vi "ArrDevMeasAction.vi"(6 "Scan":bool, 7 "DevId":i32, 8 "error in (no error)":errorcluster caption="entrée d'erreur (pas d'erreur)", 9 "CurvePointIndex":i32, 10 "AllPointIndex":i32, 11 "Device In":refnum<class "BaseDevice.lvclass"> caption="DNL_LabVIEW Object in") -> (0 "error out":errorcluster caption="sortie d'erreur", 1 "ArrDevDat":T1[](array[typedef]), 2 "ArrDevDatOut":dbl[][](array[numeric]), 3 "Device Out":refnum<class "BaseDevice.lvclass"> caption="DNL_LabVIEW Object out", 5 "MeasOut":dbl[](array[numeric]))   [LabVIEW 2019, in "BaseDevice.lvclass"]
uses:
  BaseDevice.lvclass
  Experiment Class/ArrDevData.ctl
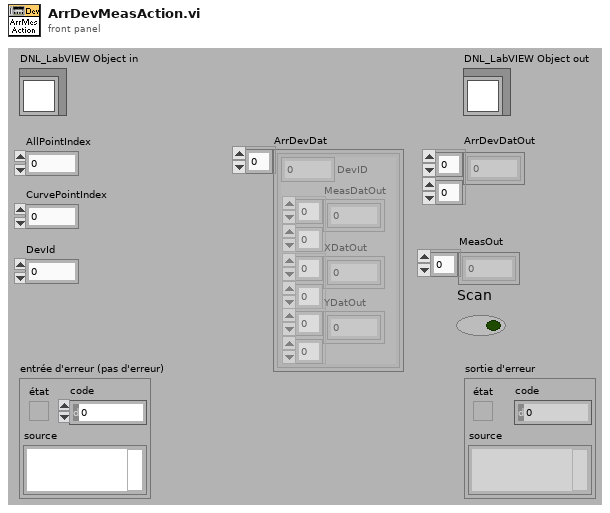
[diagram p1: front panel]
types:
  T1 = typedef "ArrDevData.ctl" = cluster{"MeasDatOut":dbl[][], "XDatOut":dbl[][], "YDatOut":dbl[][], "DevID":i32}
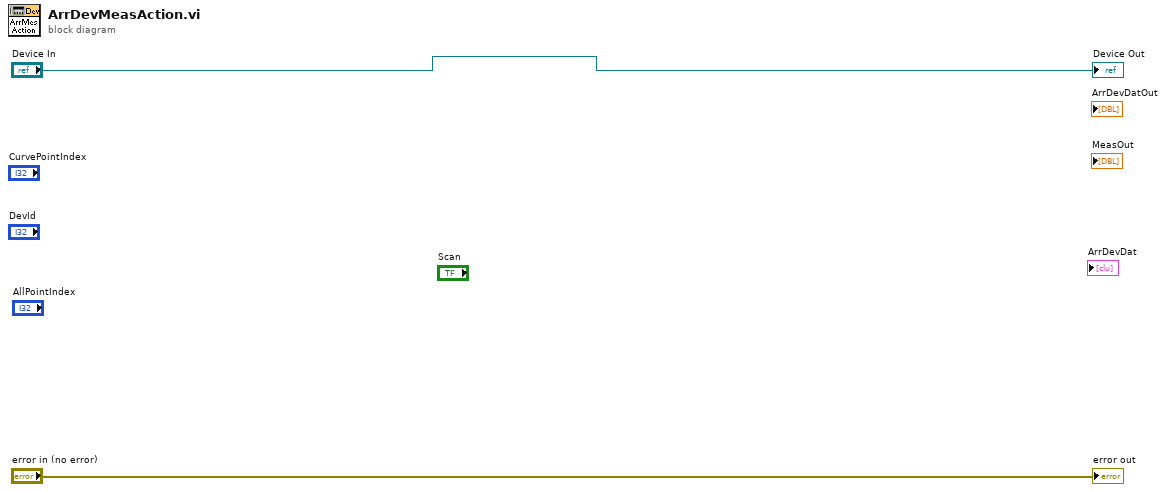
[diagram p0: block diagram]
diagram:
  "error out" <- "error in (no error)"
  "Device Out" <- "Device In"
